vi "Current Status.vi"(11 "Data Cluster in":T1) -> (0 "error out":errorcluster, 2 "Response body":string, 3 "Data Cluster out":T1)   [LabVIEW 2024, in "GUI.lvlib" / "Functions.lvlib"]
uses:
  Module Data--cluster.ctl
  <vilib>/addons/_JKI.lib/REST Client/classes/REST Client/REST Client.lvclass
  Functions.lvlib
  GUI.lvlib
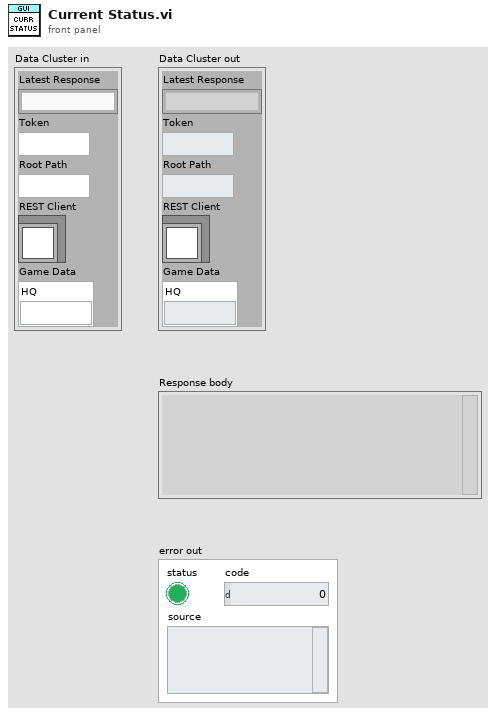
[diagram p1: front panel]
types:
  T1 = typedef "GUI.lvlib/Module Data--cluster.ctl" = cluster{"Latest Response":string, "Token":string, "Root Path":string, "REST Client":refnum<class "REST Client.lvclass">, "Game Data":cluster{"HQ":string}}
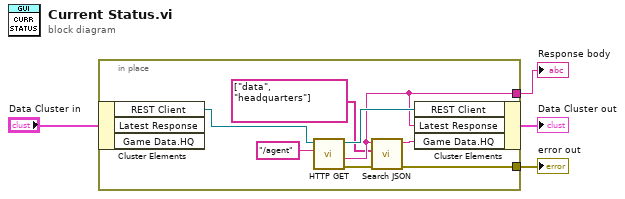
[diagram p0: block diagram]
diagram:
  n1 = in-place {
    in-place-border: [w6] -> w1
    in-place-border: [w8] -> w2
    n2 = in-place-cluster #1("Data Cluster in") -> ("REST Client"=w11:refnum<class "REST Client.lvclass">)  [unwired: 2 out]
    n3 = call-dynamic "HTTP GET.vi"("Path"="/agent", "REST Client in"=w11) -> ("error out"=w9:errorcluster, "Response body"=w8:string, "REST Client out"=w10:refnum<class "REST Client.lvclass">)  [unwired: 4 in, 3 out]
    n4 = call "Search JSON.vi"("error in"=w9, "Name Array 2"=string[] ["data", "headquarters"] ("Name Array"), "Response body"=w8) -> ("error out"=w6:errorcluster, "LabVIEW Text"=w5:string)  [unwired: 7 in]
    n5 = in-place-cluster #1("REST Client"=w10, "Latest Response"=w8, "Game Data.HQ"=w5) -> (→"Data Cluster out":T1)
  }
  "error out" <- w1
  "Response body" <- w2
